vi "COMn单步调试对话框.vi"() -> ()   [LabVIEW 2016, in "斯坦道CODMn新电路板.lvlib"]
uses:
  <vilib>/Utility/miscctls.llb/LVPointTypeDef.ctl
panel:
  in  "停止":bool
  in  "CODMn调试控件V3":cluster{"数值":u16[], "模式":enum32{"测试模式", "流程模式"}}(xcontrol)
  in  "退出":bool
  in  "启动":bool
  # "CODMn单步调试界面"
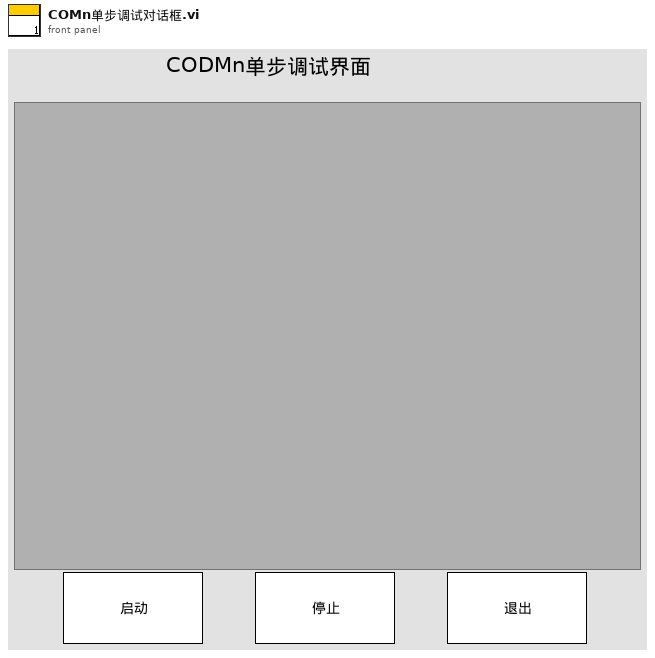
[diagram p1: front panel]
types:
  T1 = typedef "LVPointTypeDef.ctl" = cluster{"Horizontal":i16, "Vertical":i16}
  T2 = cluster{"泵类型":u8, "阀数量":u8, "纯水通道":u8, "废液通道":u8, "进样速度":u16, "出样速度":u16, "滴定速度":u16, "注射泵保温温度L":u8, "注射泵保温温度H":u8, "注射泵加热超时时间":u16, "是否存在液位检测板":u16, "A值告警下限值":u16, "A值告警上限值":u16, "B值告警下限值":u16, "B值告警上限值":u16, "AB跨度告警值":u16, "阀配置:":u8}
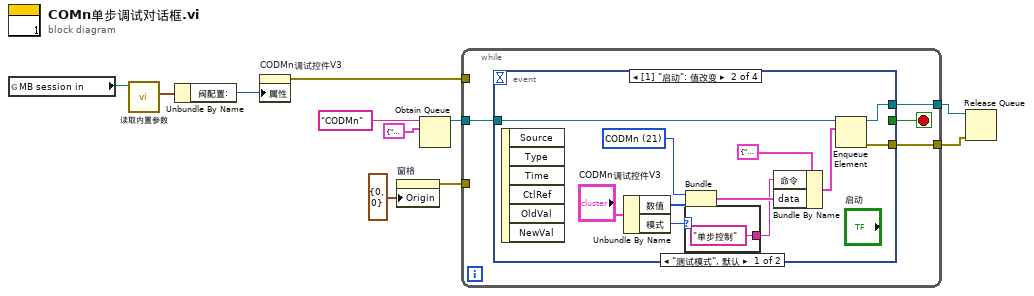
[diagram p0: block diagram]
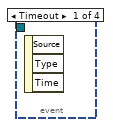
[diagram p2: hidden frame]
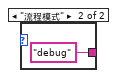
[diagram p3: hidden frame]
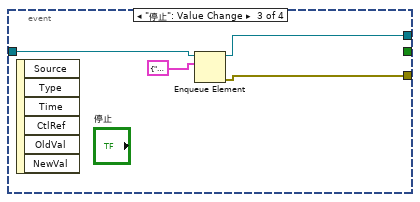
[diagram p4: hidden frame]
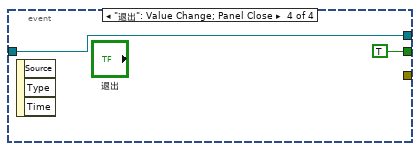
[diagram p5: hidden frame]
diagram:
  n1 = global read "VARCODMn全局变量.vi" "MB session in"() -> (w3:refnum<class "MB_Master.lvclass">)
  n2 = call "读取内置参数.vi"("MB session in"=w3) -> ("外设配置"=w2:T2)  [unwired: 6 in, 4 out]
  n3 = Unbundle By Name(w2) -> ("阀配置:"=w1:u8)
  n4 = property on="CODMn调试控件V3" class="CODMn调试控件V3 (严格)"("属性"=w1) -> (error out=w4:errorcluster)  [unwired: 2 in, 1 out]
  n5 = property on="窗格" class="Pane"("Origin"=T1 {"Horizontal"=0, "Vertical"=0} ("原点")) -> (error out=w6:errorcluster)  [unwired: 2 in, 1 out]
  n6 = Obtain Queue(name (unnamed)="CODMn" ("名称（未命名）"), element data type=cluster{"命令":string, "data":variant} {"命令"="", "data"=variant}) -> (queue out=w9:refnum<queue>)  [unwired: 3 in, 2 out]
  n7 = while {
    tunnel: w9 -> [w14]
    tunnel: [w13] -> w8
    tunnel: [w12] -> w7
    tunnel: w6 -> [_]
    tunnel: w4 -> [_]
    stop <- w15 stop-if-true
    n8 = event shown="[1] \"启动\": 值改变" {
      selector: _ -> [_ _ _ _]
      dyn-events: _ -> [_ _ _ _]
      timeout: _ -> [_ _ _ _]
      tunnel: [_ _ _ TRUE] -> w15
      tunnel: w14 -> [_ w22 w31 w33]
      tunnel: [_ w21 w30 w33] -> w13
      tunnel: [_ w20 w29 _] -> w12
      event Timeout {
        n9 = event-data() -> ()  [unwired: 1 in, 3 out]
      }
      event "启动": Value Change {
        w24 = u16 21 items=["CODMn"=21, "总磷"=1, "氨氮"=3] ("站号")
        n10 = event-data() -> ()  [unwired: 1 in, 6 out]
        n11 = Unbundle By Name("CODMn调试控件V3") -> ("数值"=w19:u16[], "模式"=w17:enum32{"测试模式", "流程模式"})
        n12 = case shown="\"测试模式\", 默认" w17 {
          tunnel: ["单步控制" ("命令") "debug" ("命令")] -> w16
          frame "测试模式", Default {
          }
          frame "流程模式" {
          }
        }
        n13 = Bundle("站号"=w24, "数值"=w19) -> (w23:cluster{"站号":u16, "数值":u16[]})  [unwired: 1 in]
        n14 = Bundle By Name(cluster=cluster{"命令":string, "data":variant} {"命令"="", "data"=variant} ("元素"), "命令"=w16, "data"=w23) -> (w25:cluster{"命令":string, "data":variant})
        n15 = Enqueue Element(queue=w22, element=w25) -> (queue out=w21:refnum<queue>, error out=w20:errorcluster)  [unwired: 2 in, 1 out]
      }
      event "停止": Value Change {
        n16 = event-data() -> ()  [unwired: 1 in, 6 out]
        n17 = Enqueue Element(queue=w31, element=cluster{"命令":string, "data":variant} {"命令"="启动", "data"=variant(cluster{"站号":u16, "控制命令":u16[]} {"站号"=21, "控制命令"=[2816]})} ("启动命令")) -> (queue out=w30:refnum<queue>, error out=w29:errorcluster)  [unwired: 2 in, 1 out]
      }
      event "退出": Value Change; Panel Close {
        n18 = event-data() -> ()  [unwired: 1 in, 3 out]
      }
    }
  }
  n19 = Release Queue(queue=w8, error in (no error)=w7) -> ()  [unwired: 1 in, 3 out]
